vi "Configure AC Current.vi"(0 "VISA resource name":refnum<visa-resource-name>, 1 "Resolution (7: 6.5 digits)":u16(ring)=7 items=["3.5 Digits"=4, "4.5 Digits"=5, "5.5 Digits"=6, "6.5 Digits"=7], 2 "Power Line Cycles (1.00)":dbl=1.0 format="%.2f", 3 "Bandwidth (300 Hz)":i32=300, 5 "error in (no error)":errorcluster, 6 "Auto Range? (T: Auto)":bool=TRUE, 7 "Digital Filter (0: Off)":u16(ring) items=["Off", "Moving Filter", "Repeating Filter"], 8 "Custom Range (0 A)":dbl format="%#_6p", 9 "Digital Filter Readings (10)":i32=10, 10 "Reference (0: Off)":u16(ring) items=["Off", "Set", "Acquire"], 12 "Reference Value (0.000 A)":dbl format="%_3g") -> (14 "VISA resource name out":refnum<visa-resource-name>, 19 "error out":errorcluster)   [LabVIEW 2020, in "Keithley 2000.lvlib"]
doc: "This VI configures the instrument to measure AC Current."
uses:
  <instrlib>/Keithley 2000/Keithley 2000.lvlib
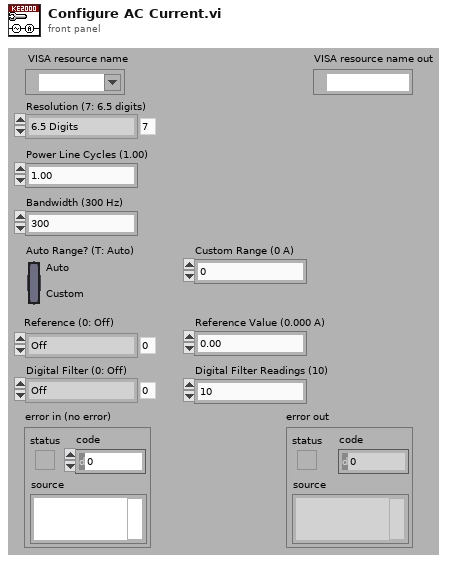
[diagram p1: front panel]
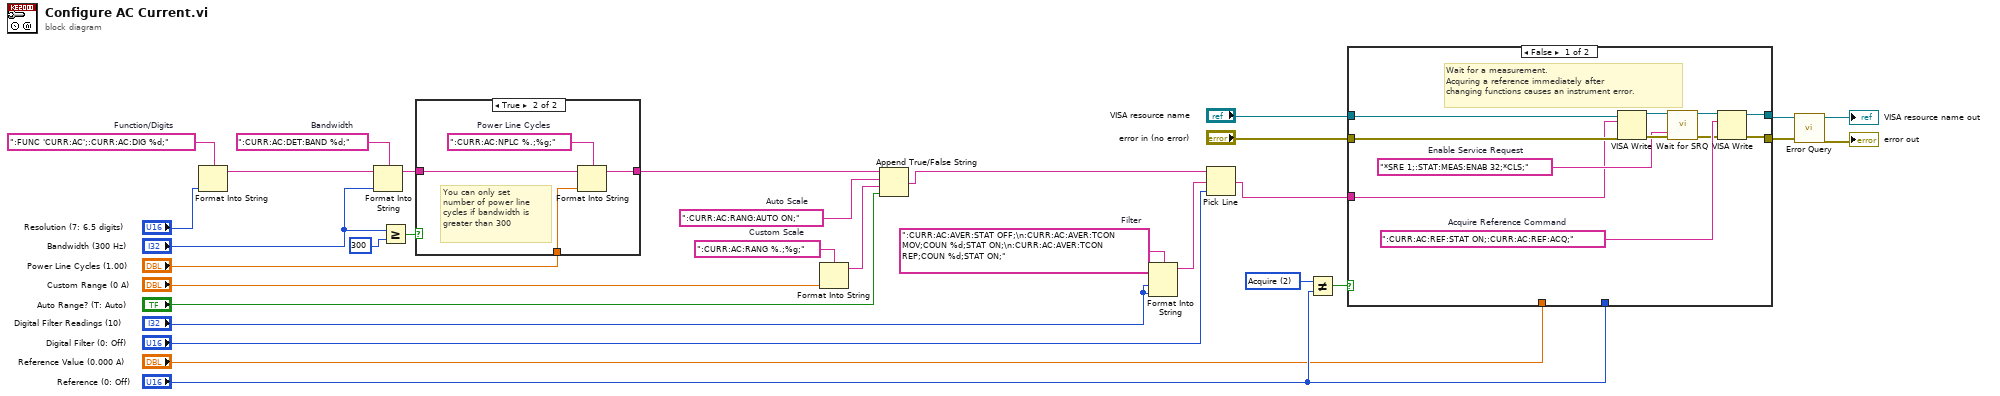
[diagram p0: block diagram]
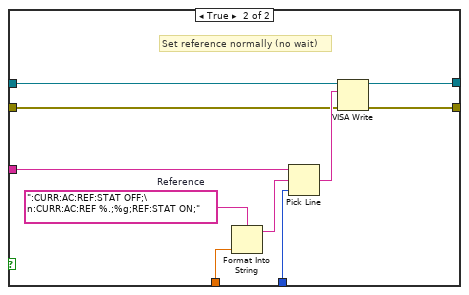
[diagram p2: hidden frame]
diagram:
  w9 = u16 2 items=["Off", "Set", "Acquire"] ("Reference (0: Off)")
  w18 = ":CURR:AC:AVER:STAT OFF;\n:CURR:AC:AVER:TCON MOV;COUN %d;STAT ON;\n:CURR:AC:AVER:TCON REP;COUN %d;STAT ON;"  # Filter
  w21 = ":CURR:AC:RANG:AUTO ON;"  # Auto Scale
  w23 = ":CURR:AC:RANG %.;%g;"  # Custom Scale
  w25 = ":CURR:AC:DET:BAND %d;"  # Bandwidth
  w26 = ":FUNC 'CURR:AC';:CURR:AC:DIG %d;"  # Function/Digits
  n1 = Format Into String(format string=w26, "Resolution (7: 6.5 digits)") -> (resulting string=w24:string)  [unwired: 2 in, 1 out]
  n2 = Format Into String(format string=w25, initial string=w24, "Bandwidth (300 Hz)") -> (resulting string=w16:string)  [unwired: 1 in, 1 out]
  n3 = Greater Or Equal?(x="Bandwidth (300 Hz)", y=300) -> (x >= y?=w13:bool)
  n4 = case shown="True" w13 {
    tunnel: "Power Line Cycles (1.00)" -> [_ w36]
    tunnel: [w32 w35] -> w28
    tunnel: w16 -> [w32 w33]
    frame False {
      # "Don't Set Power Line Cycles"
    }
    frame True {
      w34 = ":CURR:AC:NPLC %.;%g;"  # Power Line Cycles
      # "You can only set\nnumber of power line\ncycles if bandwidth is\ngreater than 300"
      n5 = Format Into String(format string=w34, initial string=w33, w36) -> (resulting string=w35:string)  [unwired: 1 in, 1 out]
    }
  }
  n6 = Format Into String(format string=w23, "Custom Range (0 A)") -> (resulting string=w22:string)  [unwired: 2 in, 1 out]
  n7 = Append True/False String(1:"Auto Range? (T: Auto)", 2:w22, 3:w21, 4:w28) -> (0:w10:string)
  n8 = Format Into String(format string=w18, "Digital Filter Readings (10)", "Digital Filter Readings (10)") -> (resulting string=w19:string)  [unwired: 2 in, 1 out]
  n9 = Pick Line(string ("")=w10, multi-line string=w19, line index="Digital Filter (0: Off)") -> (output string=w8:string)
  n10 = Not Equal?(x=w9, y="Reference (0: Off)") -> (x != y?=w5:bool)
  n11 = case shown="False" w5 {
    tunnel: "VISA resource name" -> [w44 w50]
    tunnel: "error in (no error)" -> [w45 w49]
    tunnel: "Reference Value (0.000 A)" -> [_ w55]
    tunnel: w8 -> [w37 w48]
    tunnel: [w39 w54] -> w2
    tunnel: [w40 w53] -> w1
    tunnel: "Reference (0: Off)" -> [_ w51]
    frame False {
      w38 = "*SRE 1;:STAT:MEAS:ENAB 32;*CLS;"  # Enable Service Request
      w43 = ":CURR:AC:REF:STAT ON;:CURR:AC:REF:ACQ;"  # Acquire Reference Command
      # "Wait for a measurement.\nAcquring a reference immediately after\nchanging functions causes an instrument error."
      n12 = VISA Write(VISA resource name=w44, write buffer=w37, error in (no error)=w45) -> (VISA resource name out=w47:refnum<visa-resource-name>, error out=w46:errorcluster)  [unwired: 1 out]
      n13 = call <instrlib>:"Wait for SRQ.vi"("VISA resource name"=w47, "SRQ Enable Command"=w38, "error in (no error)"=w46) -> ("VISA resource name out"=w42:refnum<visa-resource-name>, "error out"=w41:errorcluster)  [unwired: 15 in]
      n14 = VISA Write(VISA resource name=w42, write buffer=w43, error in (no error)=w41) -> (VISA resource name out=w40:refnum<visa-resource-name>, error out=w39:errorcluster)  [unwired: 1 out]
    }
    frame True {
      w57 = ":CURR:AC:REF:STAT OFF;\n:CURR:AC:REF %.;%g;REF:STAT ON;"  # Reference
      # "Set reference normally (no wait)"
      n15 = Format Into String(format string=w57, w55) -> (resulting string=w56:string)  [unwired: 2 in, 1 out]
      n16 = Pick Line(string ("")=w48, multi-line string=w56, line index=w51) -> (output string=w52:string)
      n17 = VISA Write(VISA resource name=w50, write buffer=w52, error in (no error)=w49) -> (VISA resource name out=w53:refnum<visa-resource-name>, error out=w54:errorcluster)  [unwired: 1 out]
    }
  }
  n18 = call <instrlib>:"Error Query.vi"("VISA resource name"=w1, "error in (no error)"=w2) -> ("VISA resource name out"=→"VISA resource name out":refnum<visa-resource-name>, "error out"=→"error out":errorcluster)  [unwired: 14 in, 2 out]
